vi "Check Nest Alias.vi"(7 "Actor":refnum<class "LVCAM.lvclass">, 10 "Alias":string) -> (0 "error out":errorcluster, 1 "Alias found?":bool)   [LabVIEW 2021, in "LVCAM.lvlib" / "Actor.lvclass"]
uses:
  Actor.lvclass
  LVCAM/LVCAM.lvclass
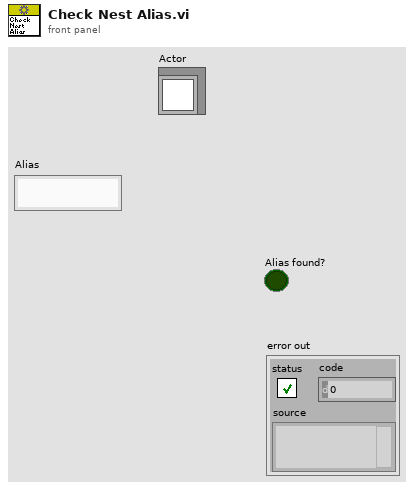
[diagram p1: front panel]
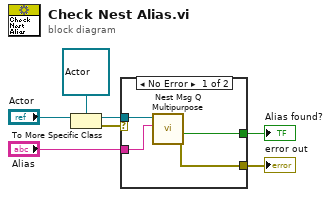
[diagram p0: block diagram]
diagram:
  n1 = To More Specific Class(target class=refnum<class "Actor.lvclass"> refnum ("LVCAM.lvlib:Self Actor.lvclass"), reference="Actor") -> (specific class reference=w5:refnum<class "Actor.lvclass">, error out=w3:errorcluster)  [unwired: 1 in]
  n2 = case shown="No Error" w3 {
    selector: w3 -> [_ w12]
    tunnel: [w9 w12] -> w7
    tunnel: w5 -> [w8 _]
    tunnel: "Alias" -> [w10 _]
    tunnel: [w11 _] -> w1
    frame No Error {
      n3 = call "Nest Msg Q Multipurpose.vi"("Alias"=w10, "Actor in"=w8) -> ("error out"=w9:errorcluster, "Alias found?"=w11:bool)  [unwired: 5 in, 3 out]
    }
    frame Error {
      # "#TypeCastError"
    }
  }
  "error out" <- w7
  "Alias found?" <- w1
